vi "FilterWheel.vi"(1 "Position set":i32=2 min=1 max=6, 2 "Serial Port":string="COM17") -> (0 "Position get":i32=2)   [LabVIEW 2018]
doc: "This example shows how to acquire a power measurement using the VIs of the driver."
uses:
  <instrlib>/Thorlabs_FW102C/Thorlabs_FW102C.lvlib
panel:
  out "OD get":dbl=0.5
  in  "OD List":dbl[](array[numeric])=[0.0, 0.5, 1.0, 2.0, 3.0, 4.0]
  out "FW error out":errorcluster
  in  "stop":bool
  out "COM Ports":string[](array[string])=["COM1", "COM3", "COM12", "COM13", "COM11", "COM10", "COM16", "COM15", "COM14", "COM17", "COM17"]
  in  "Send":bool
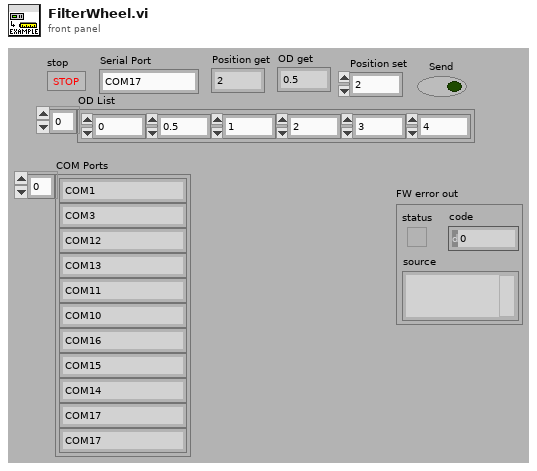
[diagram p1: front panel]
types:
  T1 = enum16{"open", "open or create", "create or replace", "create", "open (read-only)"}
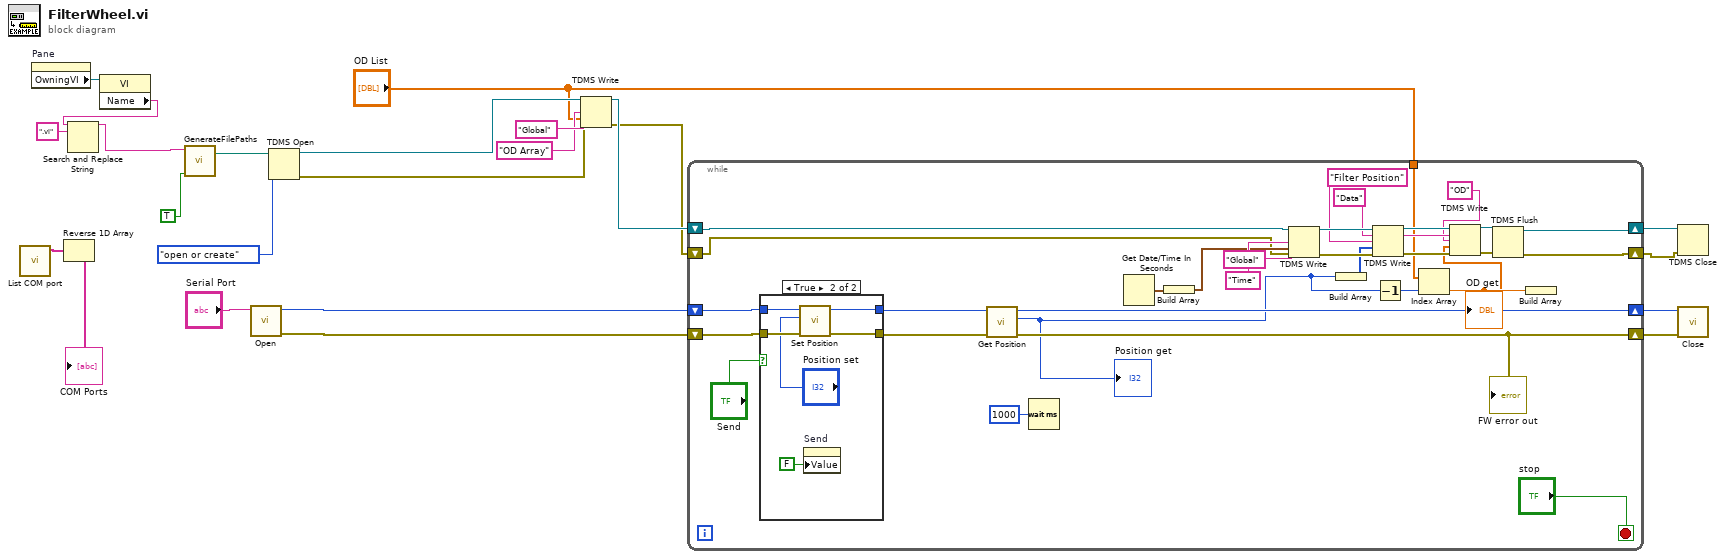
[diagram p0: block diagram]
diagram:
  n1 = call <instrlib>:"List COM port.vi"() -> ("COM Ports"=w22:string[])  [unwired: 10 in, 1 out]
  "COM Ports" <- w22
  n2 = property on="Pane" class="Pane"() -> ("OwningVI"=w16:refnum<vi>)  [unwired: 2 in, 2 out]
  n3 = Reverse 1D Array(array=w22) -> ()  [unwired: 1 out]
  n4 = property class="VI"(reference=w16) -> ("Name"=w10:string)  [unwired: 1 in, 2 out]
  n5 = Search and Replace String(input string=w10, search string=".vi") -> (result string=w14:string)  [unwired: 6 in, 3 out]
  n6 = call "GenerateFilePaths.vi"("Logfile? (F)"=TRUE ("Logfile?"), "Device Name"=w14) -> ("Path"=w12:path)  [unwired: 3 in]
  n7 = call <instrlib>:"Open.vi"("Serial Port"="Serial Port") -> ("error out"=w20:errorcluster, "FW102C out"=w21:i32)  [unwired: 8 in, 1 out]
  n8 = TDMS Open(10:T1."open or create" ("operation (0:open)"), 11:w12) -> (0:w4:errorcluster, 3:w5:refnum<k34>)  [unwired: 5 in]
  n9 = TDMS Write(0:w5, 5:"Global" ("group name in (Untitled)"), 7:"OD Array" ("group name in (Untitled)"), 9:"OD List", 11:w4) -> (4:w3:refnum<k34>, 15:w2:errorcluster)  [unwired: 1 in, 2 out]
  n10 = while {
    shift-right: [w50] -> w18
    shift-left: w21 -> [w55]
    shift-right: [w51] -> w19
    shift-left: w20 -> [w54]
    shift-right: [w36] -> w9
    shift-left: w3 -> [w43]
    shift-right: [w35] -> w8
    shift-left: w2 -> [w41]
    tunnel: "OD List" -> [w28]
    stop <- "stop" stop-if-true
    n11 = case shown="True" "Send" {
      tunnel: w55 -> [w57 w63]
      tunnel: w54 -> [w56 w62]
      tunnel: [w57 w61] -> w53
      tunnel: [w56 w60] -> w52
      frame False {
      }
      frame True {
        n12 = call <instrlib>:"Set Position.vi"("error in (no error)"=w62, "Position"="Position set", "FW102C in"=w63) -> ("error out"=w60:errorcluster, "FW102C out"=w61:i32)  [unwired: 7 in]
        n13 = property on="Send" class="Bool (strict)"("Value"=FALSE ("Send")) -> ()  [unwired: 2 in, 2 out]
      }
    }
    n14 = call <instrlib>:"Get Position.vi"("error in (no error)"=w52, "FW102C in"=w53) -> ("error out"=w51:errorcluster, "Position"=w24:i32, "FW102C out"=w50:i32)  [unwired: 7 in]
    "Position get" <- w24
    "FW error out" <- w51
    n15 = Wait (ms)(milliseconds to wait=u32 1000) -> ()  [unwired: 1 out]
    n16 = Get Date/Time In Seconds() -> (seconds since 1Jan1904=w46:timestamp)
    n17 = Build Array(w46) -> (w44:timestamp[])
    n18 = TDMS Write(0:w43, 5:"Global" ("group name in (Untitled)"), 7:"Time" ("group name in (Untitled)"), 9:w44, 11:w41) -> (4:w42:refnum<k34>, 15:w40:errorcluster)  [unwired: 1 in, 2 out]
    n19 = Build Array(w24) -> (w39:i32[])
    n20 = TDMS Write(0:w42, 5:"Data" ("group name in (Untitled)"), 7:"Filter Position" ("group name in (Untitled)"), 9:w39, 11:w40) -> (4:w33:refnum<k34>, 6:w32:string, 15:w31:errorcluster)  [unwired: 1 in, 1 out]
    n21 = Decrement(x=w24) -> (x-1=w23:i32)
    n22 = Index Array(array=w28, index=w23) -> (element=w27:dbl)
    "OD get" <- w27
    n23 = Build Array(w27) -> (w26:dbl[])
    n24 = TDMS Write(0:w33, 5:w32, 7:"OD" ("group name in (Untitled)"), 9:w26, 11:w31) -> (4:w30:refnum<k34>, 15:w29:errorcluster)  [unwired: 1 in, 2 out]
    n25 = TDMS Flush(4:w29, 7:w30) -> (0:w35:errorcluster, 3:w36:refnum<k34>)
  }
  n26 = TDMS Close(8:w8, 11:w9) -> ()  [unwired: 2 out]
  n27 = call <instrlib>:"Close.vi"("error in (no error)"=w19, "FW102C in"=w18) -> ()  [unwired: 9 in, 1 out]
